vi "Load Keys.vi"(8 "error in (no error)":errorcluster, 11 "[MV] Key Generator in":refnum<class "[MV] Key Generator.lvclass">) -> (0 "error out":errorcluster, 3 "[MV] Key Generator out":refnum<class "[MV] Key Generator.lvclass">)   [LabVIEW 2020, in "[MV] Key Generator.lvlib" / "[MV] Key Generator.lvclass"]
uses:
  [MV] Key Generator.lvclass
  <vilib>/YU/YU_Encrypt/AES/AES.lvclass
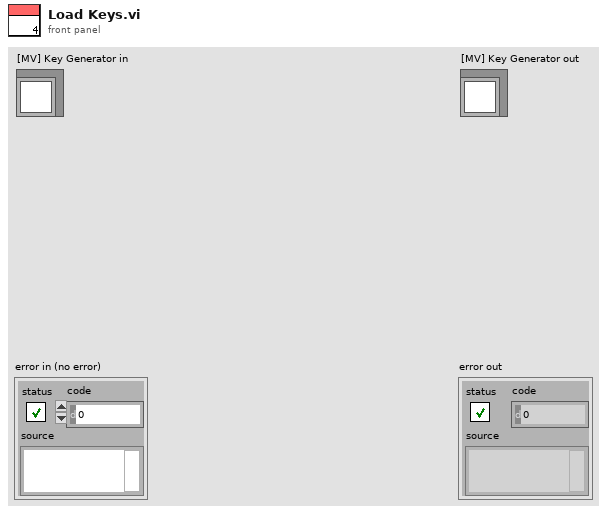
[diagram p1: front panel]
types:
  T1 = enum16{"open", "replace", "create", "open or create", "replace or create", "replace or create with confirmation"}
  T2 = map{string, cluster{"private":string, "public":string}}
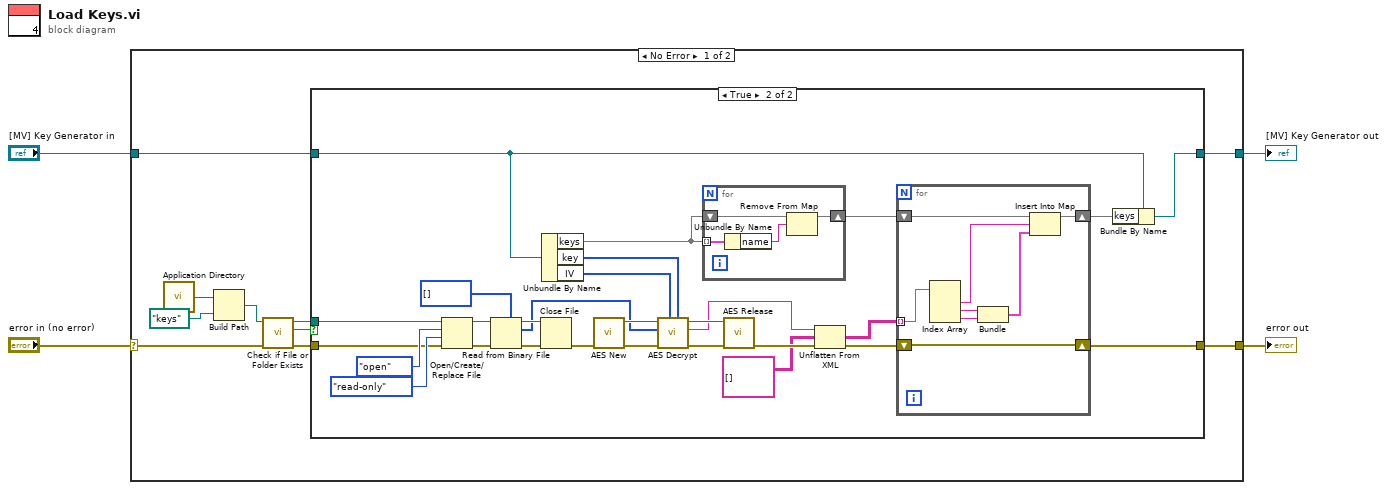
[diagram p0: block diagram]
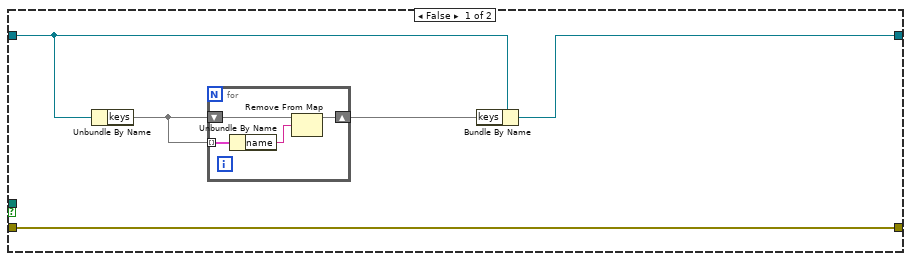
[diagram p2: hidden frame]
diagram:
  n1 = case shown="No Error" "error in (no error)" {
    selector: "error in (no error)" -> [w12 w65]
    tunnel: [w5 w65] -> w3
    tunnel: [w6 w64] -> w1
    tunnel: "[MV] Key Generator in" -> [w7 w64]
    frame No Error {
      n2 = call <vilib>:"Application Directory.vi"() -> ("Application Directory"=w13:path)
      n3 = Build Path(base path=w13, name or relative path=path "keys") -> (appended path=w11:path)
      n4 = call <vilib>:"Check if File or Folder Exists.vi"("error in (no error)"=w12, "path"=w11) -> ("error out"=w9:errorcluster, "file or folder exists?"=w10:bool, "dup path"=w8:path)  [unwired: 7 in]
      n5 = case shown="True" w10 {
        tunnel: w9 -> [w18 w44]
        tunnel: w8 -> [_ w43]
        tunnel: w7 -> [w17 w29]
        tunnel: [w15 w28] -> w6
        tunnel: [w18 w27] -> w5
        frame False {
          n6 = Unbundle By Name(w17) -> ("keys"=w19:T2)
          n7 = for {
            tunnel: w19 -> [w23] mode=indexing
            shift-right: [w20] -> w16
            shift-left: w19 -> [w22]
            n8 = Unbundle By Name(w23) -> ("name"=w21:string)
            n9 = Remove From Map(10:w21, 11:w22) -> (3:w20:T2)  [unwired: 2 out]
          }
          n10 = Bundle By Name(cluster=w17, "keys"=w16) -> (w15:refnum<class "[MV] Key Generator.lvclass">)
        }
        frame True {
          n11 = Open/Create/Replace File(file path (use dialog)=w43, error in=w44, operation (0:open)=T1."open", access (0:read/write)=enum16{"read/write", "read-only", "write-only"}."read-only") -> (refnum out=w49:refnum<file>, error out=w48:errorcluster)  [unwired: 2 in, 1 out]
          n12 = Read from Binary File(5:u8[] [] ("encrypted"), 8:w48, 11:w49) -> (0:w46:errorcluster, 2:w25:u8[], 3:w47:refnum<file>)  [unwired: 3 in, 1 out]
          n13 = Close File(refnum=w47, error in=w46) -> (error out=w26:errorcluster)  [unwired: 1 out]
          n14 = Unbundle By Name(w29) -> ("keys"=w36:T2, "key"=w41:u8[], "IV"=w40:u8[])
          n15 = call <vilib>:"AES New.vi"("error in (no error)"=w26) -> ("error out"=w42:errorcluster, "AES out"=w39:refnum<class "AES.lvclass">)  [unwired: 9 in]
          n16 = call <vilib>:"AES Decrypt.vi"("Key"=w41, "IV"=w40, "error in (no error)"=w42, "encrypted_data"=w25, "AES in"=w39) -> ("error out"=w38:errorcluster, "data"=w34:string, "AES out"=w37:refnum<class "AES.lvclass">)  [unwired: 4 in]
          n17 = for {
            tunnel: w36 -> [w63] mode=indexing
            shift-right: [w60] -> w32
            shift-left: w36 -> [w62]
            n18 = Unbundle By Name(w63) -> ("name"=w61:string)
            n19 = Remove From Map(10:w61, 11:w62) -> (3:w60:T2)  [unwired: 2 out]
          }
          n20 = call <vilib>:"AES Release.vi"("error in (no error)"=w38, "AES in"=w37) -> ("error out"=w35:errorcluster)  [unwired: 9 in]
          n21 = Unflatten From XML(xml string=w34, type=string[][] [], error in (no error)=w35) -> (value=w31:string[][], error out=w24:errorcluster)
          n22 = for {
            shift-right: [w55] -> w30
            shift-left: w32 -> [w56]
            tunnel: w31 -> [w57] mode=indexing
            shift-right: [w52] -> w27
            shift-left: w24 -> [w52]
            n23 = Index Array(array=w57) -> (element #1=w54:string, element #2=w58:string, element #3=w59:string)  [unwired: 3 in]
            n24 = Bundle("public"=w58, "public"=w59) -> (w53:cluster{"public":string, "public":string})  [unwired: 1 in]
            n25 = Insert Into Map(map in=w56, key=w54, value=w53) -> (map out=w55:T2)  [unwired: 2 out]
          }
          n26 = Bundle By Name(cluster=w29, "keys"=w30) -> (w28:refnum<class "[MV] Key Generator.lvclass">)
        }
      }
    }
    frame Error {
    }
  }
  "error out" <- w3
  "[MV] Key Generator out" <- w1
